vi "merge_errors.vi"   [LabVIEW 2015]
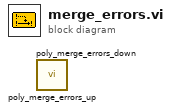
[diagram p0: block diagram]
diagram:
  n1 = call "poly_merge_errors_up.vi"() -> ()  [unwired: 11 in, 1 out]
  n2 = call "poly_merge_errors_down.vi"() -> ()  [unwired: 11 in, 1 out]
